vi "PlyTrgChange.vi"   [LabVIEW 2013]
uses:
  Multiplexer_Opmux.lvclass
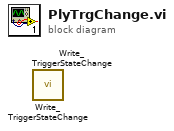
[diagram p0: block diagram]
diagram:
  n1 = call-dynamic "Write_TriggerStateChange.vi"() -> ()  [unwired: 10 in, 2 out]
  n2 = call-dynamic "Write_TriggerStateChange.vi"() -> ()  [unwired: 10 in, 2 out]
